vi "_RT_CtrlLoop_ResourcesMonitor.vi"(8 "error in (no error)":errorcluster, 10 "system state":refnum<data-value>) -> (0 "error out":errorcluster)   [LabVIEW 2018]
uses:
  PublicSubVI/Ctl/_ctl_RT_System_State.ctl
  <vilib>/nisyscfg/Close (System).vi
  <vilib>/nisyscfg/nisyscfg.lvlib
  <resource>/objmgr/nisysapi.rc
  <vilib>/NI_Real-Time Target Support.lvlib
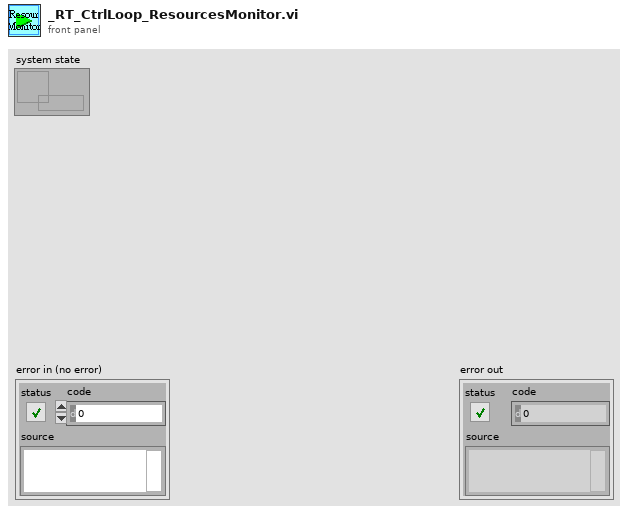
[diagram p1: front panel]
types:
  T1 = typedef "_ctl_RT_System_State.ctl" = enum16{"initialize", "idle", "working", "disconnect"}
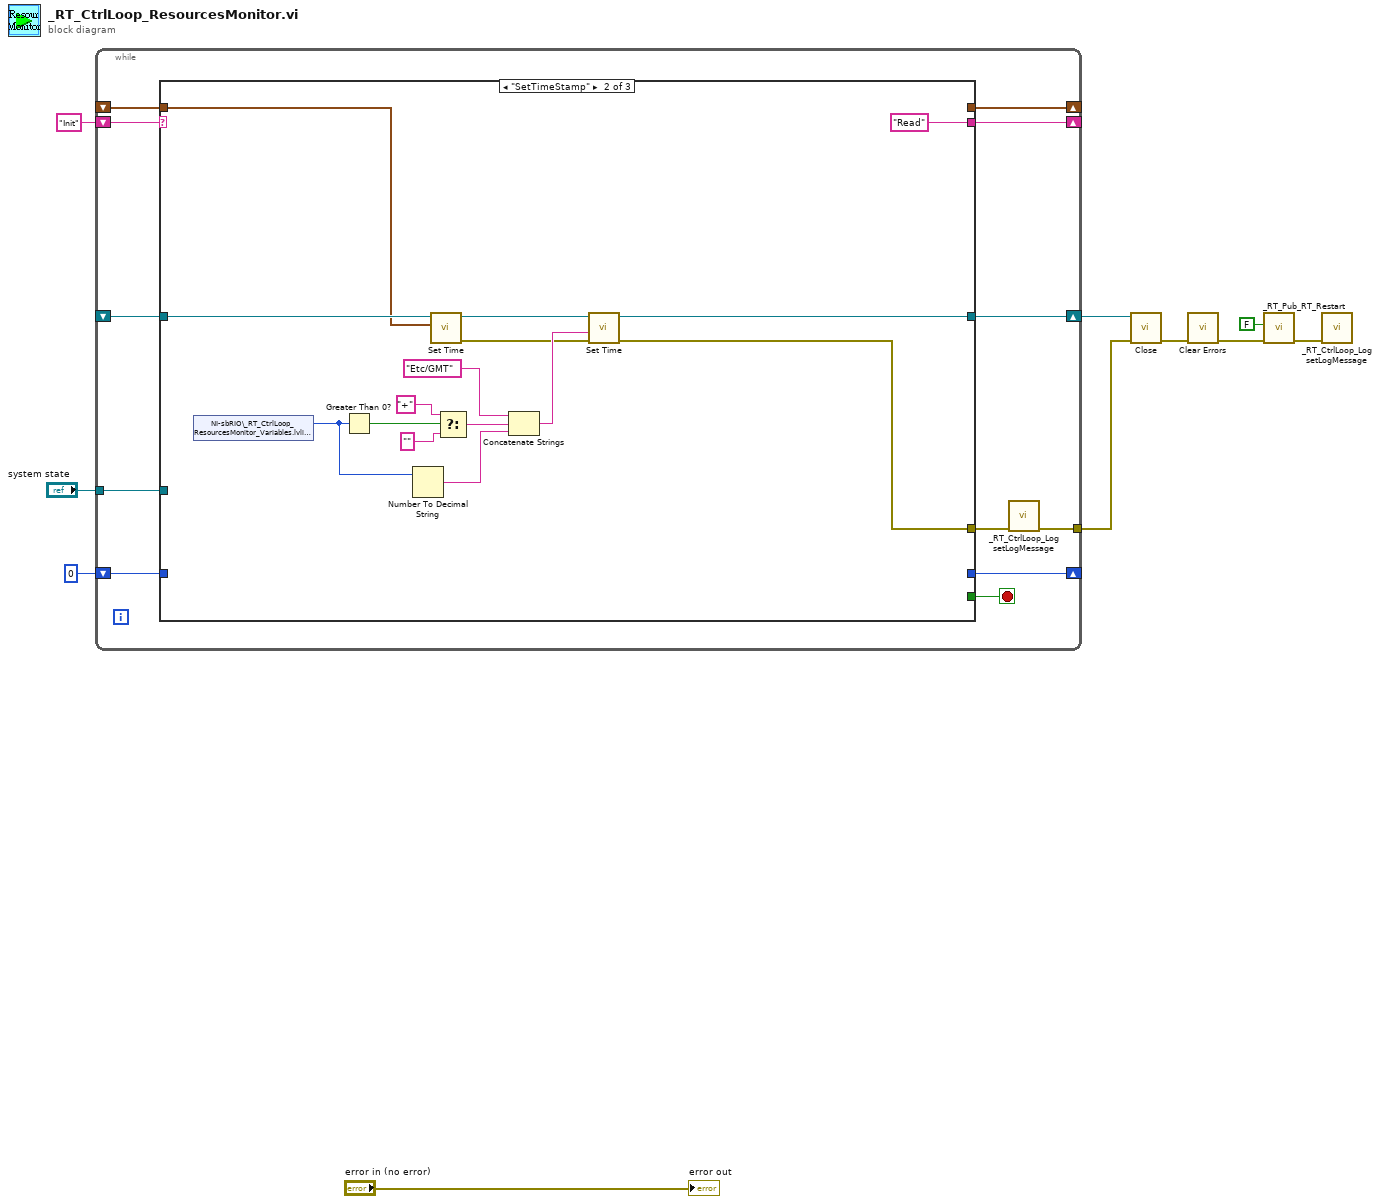
[diagram p0: block diagram]
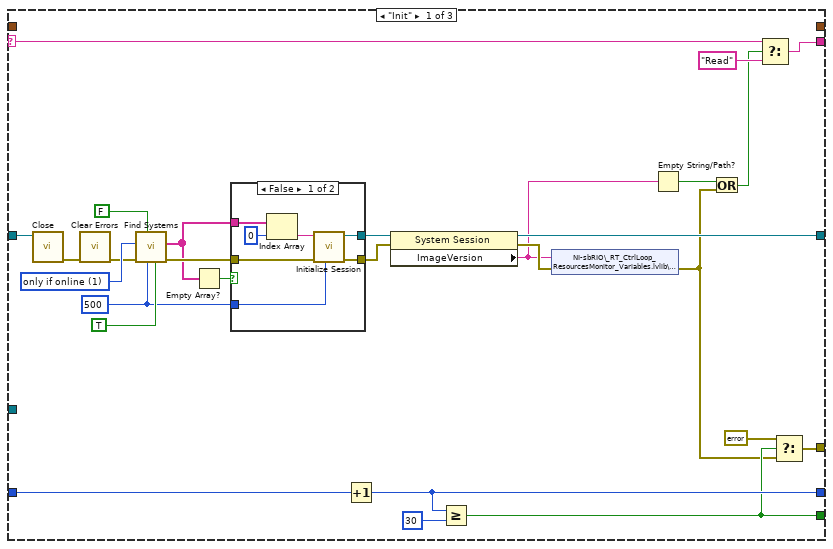
[diagram p2: hidden frame]
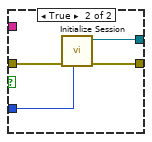
[diagram p3: hidden frame]
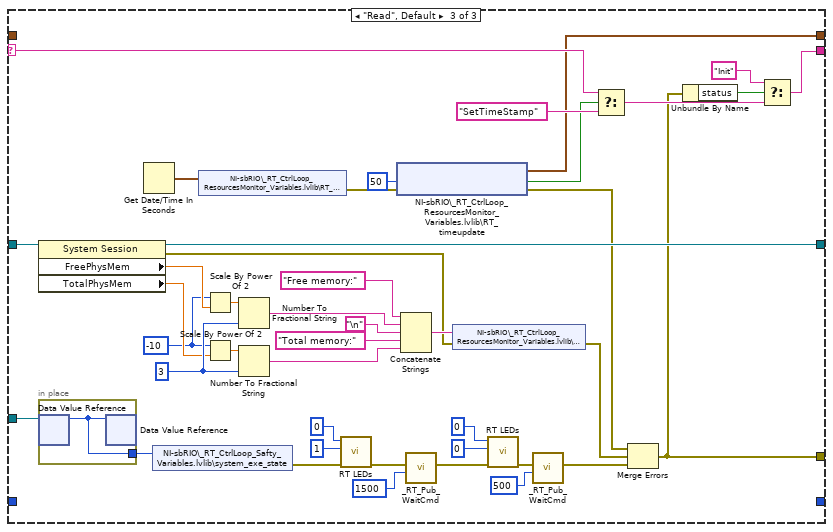
[diagram p4: hidden frame]
diagram:
  n1 = while {
    shift-right: [w15] -> _
    shift-left: "Init" -> [w22]
    shift-right: [w21] -> w7
    shift-left: _ -> [w20]
    shift-right: [w19] -> _
    shift-left: _ -> [w18]
    tunnel: "system state" -> [w14]
    shift-right: [w16] -> _
    shift-left: 0 -> [w17]
    tunnel: [w11] -> w2
    stop <- w12 stop-if-true
    n2 = case shown="\"SetTimeStamp\"" w22 {
      selector: w22 -> [w40 _ w106]
      tunnel: [w43 w74 w117] -> w21
      tunnel: [w48 "Read" w115] -> w15
      tunnel: w20 -> [w45 w65 w89]
      tunnel: [_ _ w83] -> w19
      tunnel: w18 -> [_ w64 _]
      tunnel: w17 -> [w46 _ _]
      tunnel: [w38 _ _] -> w16
      tunnel: [w36 w73 w76] -> w13
      tunnel: w14 -> [_ _ w88]
      tunnel: [w35 _ _] -> w12
      frame "Init" {
        w27 = u32 500 ("Timeout (4000 ms)")
        w32 = u32 1 items=["none"=0, "only if online"=1, "all"=3] ("Include Cached Results (all)")
        n3 = call-poly <vilib>:"Close.vi"("Session in"=w45) -> ("error out"=w49:errorcluster)  [unwired: 10 in]
        n4 = call <vilib>:"Clear Errors.vi"("error in (no error)"=w49) -> ("error out"=w31:errorcluster)  [unwired: 5 in, 1 out]
        n5 = call <vilib>:"Find Systems.vi"("Only Installable Systems (F)"=TRUE, "Timeout (4000 ms)"=w27, "Detect Online Systems (T)"=FALSE, "error in (no error)"=w31, "Include Cached Results (all)"=w32) -> ("error out"=w30:errorcluster, "Detected Systems"=w28:string[])  [unwired: 4 in, 1 out]
        n6 = Empty Array?(array=w28) -> (empty?=w29:bool)
        n7 = case shown="False" w29 {
          tunnel: [w56 w60] -> w44
          tunnel: [w55 w59] -> w41
          tunnel: w30 -> [w54 w58]
          tunnel: w28 -> [w52 _]
          tunnel: w27 -> [w50 w57]
          frame False {
            n8 = Index Array(array=w52, index=0) -> (element=w51:string)
            n9 = call <vilib>:"Initialize Session.vi"("Connect Timeout (4000 ms)"=w50, "error in (no error)"=w54, "Target (localhost)"=w51) -> ("error out"=w55:errorcluster, "Session out"=w56:refnum<k21>)  [unwired: 7 in]
          }
          frame True {
            n10 = call <vilib>:"Initialize Session.vi"("Connect Timeout (4000 ms)"=w57, "error in (no error)"=w58) -> ("error out"=w59:errorcluster, "Session out"=w60:refnum<k21>)  [unwired: 8 in]
          }
        }
        n11 = Increment(x=w46) -> (x+1=w38:i32)
        n12 = property class="System Session"(reference=w44, error in=w41) -> (reference out=w43:refnum<k21>, error out=w42:errorcluster, "ImageVersion"=w23:string)
        n13 = Greater Or Equal?(x=w38, y=30) -> (x >= y?=w35:bool)
        n14 = shared-variable "NI-sbRIO\\_RT_CtrlLoop_ResourcesMonitor_Variables.lvlib\\SystemVersion"(w23, error in=w42) -> (error out=w24:errorcluster)
        n15 = Empty String/Path?(string/path=w23) -> (empty?=w26:bool)
        n16 = Or(x=w26, y=w24) -> (x .or. y?=w25:bool)
        n17 = Select(t=w40, s=w25, f="Read") -> (s? t:f=w48:string)
        n18 = Select(t=errorcluster {"status"=TRUE, "code"=5001, "source"="Resources Time Out"} ("error out"), s=w35, f=w24) -> (s? t:f=w36:errorcluster)
      }
      frame "SetTimeStamp" {
        n19 = shared-variable "NI-sbRIO\\_RT_CtrlLoop_ResourcesMonitor_Variables.lvlib\\RT TimeZone"() -> (w61:i32)  [unwired: 1 in, 1 out]
        n20 = Greater Than 0?(x=w61) -> (x > 0?=w69:bool)
        n21 = Number To Decimal String(number=w61) -> (decimal integer string=w67:string)  [unwired: 1 in]
        n22 = call <vilib>:"Set Time.vi"("Time"=w64, "Session in (localhost)"=w65) -> ("error out"=w62:errorcluster, "Session out"=w63:refnum<k21>)  [unwired: 6 in, 2 out]
        n23 = Select(t="+", s=w69, f="") -> (s? t:f=w72:string)
        n24 = Concatenate Strings("Etc/GMT" ("String"), w72, w67) -> (w66:string)
        n25 = call <vilib>:"Set Time.vi"("error in (no error)"=w62, "Time Zone"=w66, "Session in (localhost)"=w63) -> ("error out"=w73:errorcluster, "Session out"=w74:refnum<k21>)  [unwired: 5 in, 2 out]
      }
      frame "Read", Default {
        w99 = i16 -10 ("n")
        w114 = i16 3 ("precision (6)")
        n26 = property class="System Session"(reference=w89) -> (reference out=w117:refnum<k21>, error out=w79:errorcluster, "FreePhysMem"=w103:dbl, "TotalPhysMem"=w100:dbl)  [unwired: 1 in]
        n27 = in-place {
          in-place-border: [w118] -> w87
          n28 = in-place-dvr #1(w88) -> (w118:T1)  [unwired: 1 out]
          n29 = in-place-dvr #1(w118) -> ()  [unwired: 2 out]
        }
        n30 = Get Date/Time In Seconds() -> (seconds since 1Jan1904=w84:timestamp)
        n31 = shared-variable "NI-sbRIO\\_RT_CtrlLoop_Safty_Variables.lvlib\\system_exe_state"(w87) -> (error out=w86:errorcluster)  [unwired: 1 in]
        n32 = shared-variable "NI-sbRIO\\_RT_CtrlLoop_ResourcesMonitor_Variables.lvlib\\RT_SysTimeStamp"(w84) -> (error out=w82:errorcluster)  [unwired: 1 in]
        n33 = Scale By Power Of 2(n=w99, x=w103) -> (x*2^n=w102:dbl)
        n34 = Scale By Power Of 2(n=w99, x=w100) -> (x*2^n=w101:dbl)
        n35 = Number To Fractional String(number=w102, precision (6)=w114) -> (F-format string=w111:string)  [unwired: 2 in]
        n36 = Number To Fractional String(number=w101, precision (6)=w114) -> (F-format string=w109:string)  [unwired: 2 in]
        n37 = call <vilib>:"RT LEDs.vi"("error in (no error)"=w86, "State"=1, "LED Num"=0) -> ("error out"=w96:errorcluster)  [unwired: 3 in, 1 out]
        n38 = shared-variable "NI-sbRIO\\_RT_CtrlLoop_ResourcesMonitor_Variables.lvlib\\RT_timeupdate"(error in=w82, 50 ("ms timeout (0)")) -> (w83:timestamp, error out=w77:errorcluster, w81:bool)
        n39 = Concatenate Strings("Free memory:", w111, "\n", "Total memory:", w109) -> (w113:string)
        n40 = call "_RT_Pub_WaitCmd.vi"("milliseconds to wait"=u32 1500, "error in (no error)"=w96) -> ("error out"=w92:errorcluster)  [unwired: 9 in]
        n41 = shared-variable "NI-sbRIO\\_RT_CtrlLoop_ResourcesMonitor_Variables.lvlib\\ResourceUsage"(w113, error in=w79) -> (error out=w78:errorcluster)
        n42 = call <vilib>:"RT LEDs.vi"("error in (no error)"=w92, "State"=0, "LED Num"=0) -> ("error out"=w90:errorcluster)  [unwired: 3 in, 1 out]
        n43 = call "_RT_Pub_WaitCmd.vi"("milliseconds to wait"=u32 500, "error in (no error)"=w90) -> ("error out"=w85:errorcluster)  [unwired: 9 in]
        n44 = Select(t=w106, s=w81, f="SetTimeStamp") -> (s? t:f=w104:string)
        n45 = Merge Errors(w77, w78, w85) -> (w76:errorcluster)
        n46 = Unbundle By Name(w76) -> ("status"=w116:bool)
        n47 = Select(t="Init", s=w116, f=w104) -> (s? t:f=w115:string)
      }
    }
    n48 = call "_RT_CtrlLoop_Log setLogMessage.vi"("error in"=w13) -> ("error out"=w11:errorcluster)  [unwired: 9 in, 1 out]
  }
  n49 = call-poly <vilib>:"Close.vi"("error in (no error)"=w2, "Session in"=w7) -> ("error out"=w6:errorcluster)  [unwired: 9 in]
  n50 = call <vilib>:"Clear Errors.vi"("error in (no error)"=w6) -> ("error out"=w4:errorcluster)  [unwired: 5 in, 1 out]
  n51 = call "_RT_Pub_RT_Restart.vi"("error in (no error)"=w4, "Safe Mode?"=FALSE) -> ("error out"=w1:errorcluster)  [unwired: 9 in]
  n52 = call "_RT_CtrlLoop_Log setLogMessage.vi"("error in"=w1) -> ()  [unwired: 9 in, 2 out]
  "error out" <- "error in (no error)"
